vi "Get Channel Data.vi"(8 "error in":errorcluster, 11 "Channel Ref in":refnum<data-value>) -> (0 "error out":errorcluster, 2 "Channel Data":T1, 3 "Channel Ref out":refnum<data-value>)   [LabVIEW 2024, in "Config File Parser.lvlib" / "Channel.lvclass"]
uses:
  Channel.lvclass
  Channel.lvclass/Channel.ctl
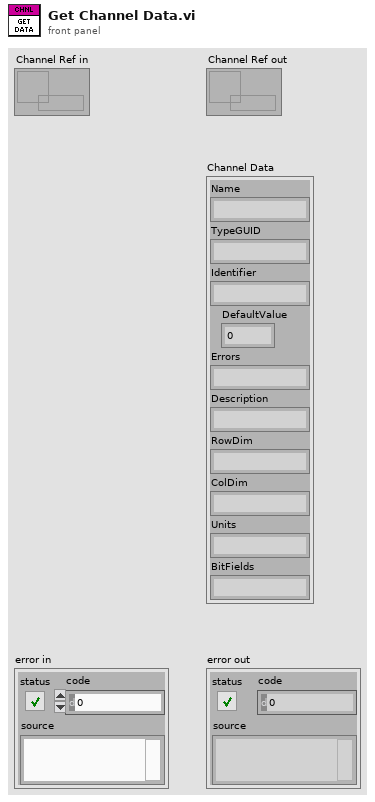
[diagram p1: front panel]
types:
  T1 = cluster{"Name":string, "TypeGUID":string, "Identifier":string, "DefaultValue":dbl, "Errors":string, "Description":string, "RowDim":string, "ColDim":string, "Units":string, "BitFields":string}
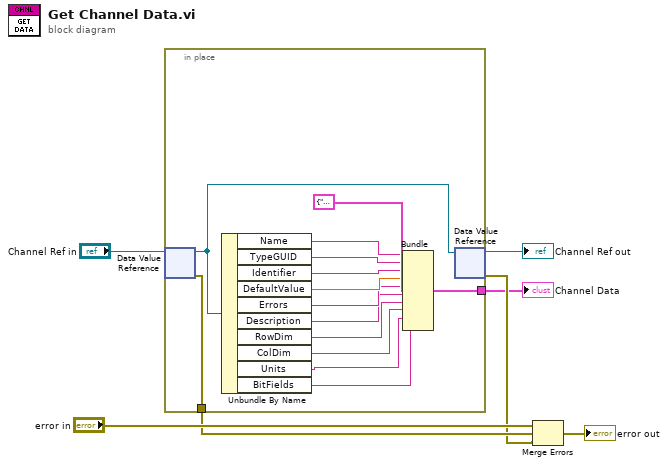
[diagram p0: block diagram]
diagram:
  n1 = in-place {
    in-place-border: [w9] -> w1
    in-place-border: [w21] -> w6
    n2 = in-place-dvr #1("Channel Ref in") -> (w8:refnum<class "Channel.lvclass">, w21:errorcluster)
    n3 = Unbundle By Name(w8) -> ("Name"=w19:string, "TypeGUID"=w18:string, "Identifier"=w17:string, "DefaultValue"=w16:dbl, "Errors"=w15:string, "Description"=w14:string, "RowDim"=w13:string, "ColDim"=w12:string, "Units"=w11:string, "BitFields"=w10:string)
    n4 = Bundle(cluster=T1 {"Name"="", "TypeGUID"="", "Identifier"="", "DefaultValue"=0.0, "Errors"="", "Description"="", "RowDim"="", "ColDim"="", "Units"="", "BitFields"=""}, "Name"=w19, "TypeGUID"=w18, "Identifier"=w17, "DefaultValue"=w16, "Errors"=w15, "Description"=w14, "RowDim"=w13, "ColDim"=w12, "Units"=w11, "BitFields"=w10) -> (w9:T1)
    n5 = in-place-dvr #1(w8) -> (→"Channel Ref out":refnum<data-value>, w5:errorcluster)
  }
  "Channel Data" <- w1
  n6 = Merge Errors("error in", w6, w5) -> (→"error out":errorcluster)
